vi "powerSource (1).vi"() -> ()   [LabVIEW 2013]
panel:
  out "Current, A":string
  in  "VISA Address":refnum<visa-resource-name>
  out "Voltage, V":string
  in  "Set Current":bool
  in  "Current":dbl
  in  "Set Voltage":bool
  in  "Voltage":dbl
  in  "Display Mode":enum32{"Normal", "Waveform", "Dial"}(radio)
  in  "Channel 2":bool
  out "Return":string
  in  "SCPI Command":string
  in  "Exit":bool
  in  "Read":bool
  in  "Write":bool
  in  "Connect":bool
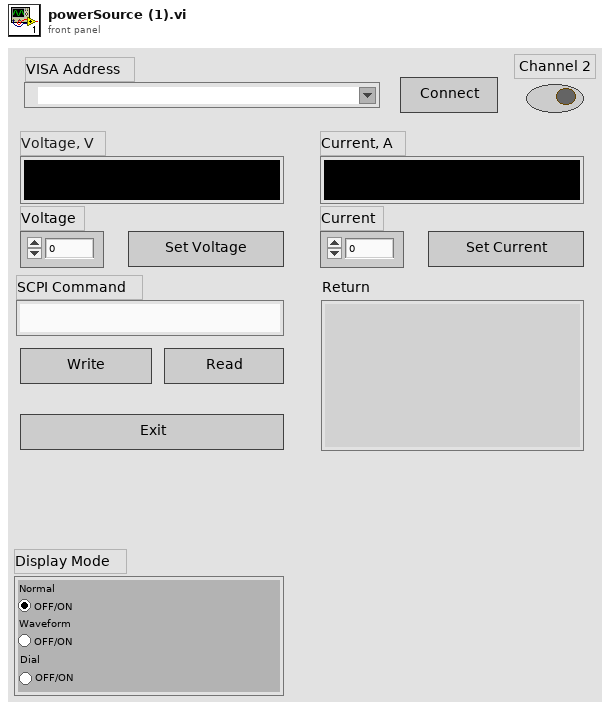
[diagram p1: front panel]
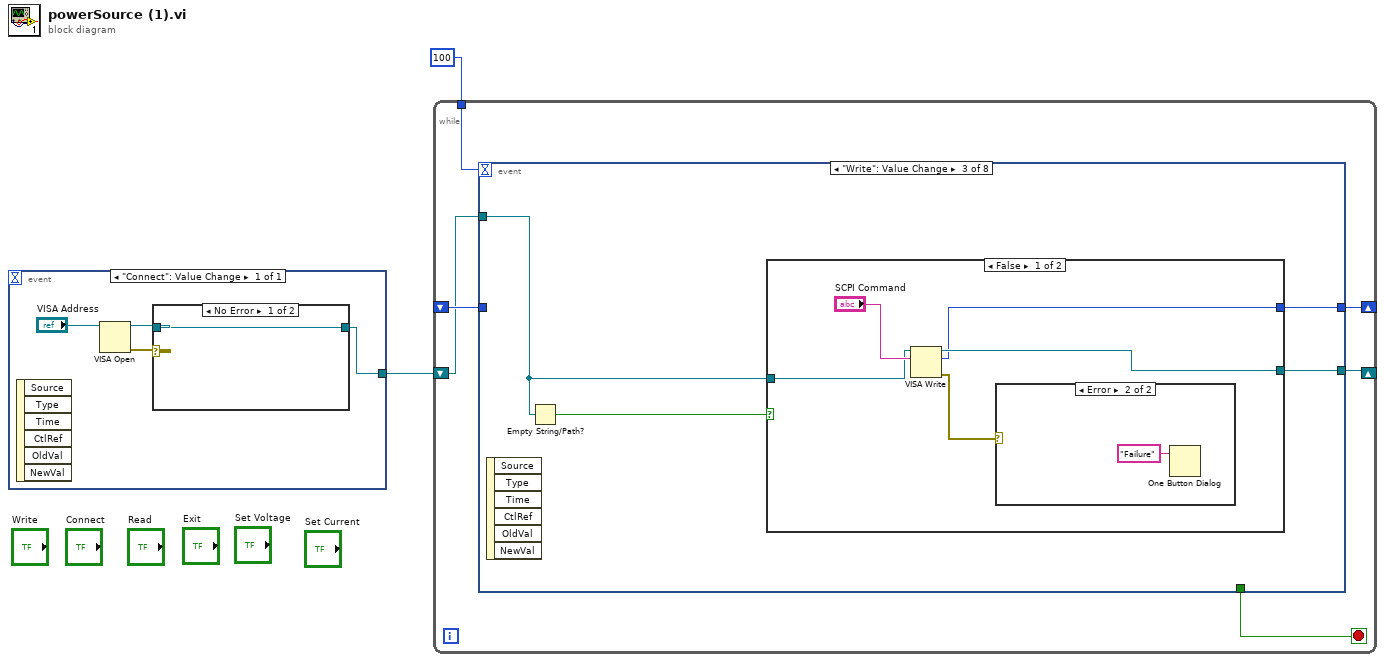
[diagram p0: block diagram]
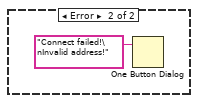
[diagram p2: hidden frame]
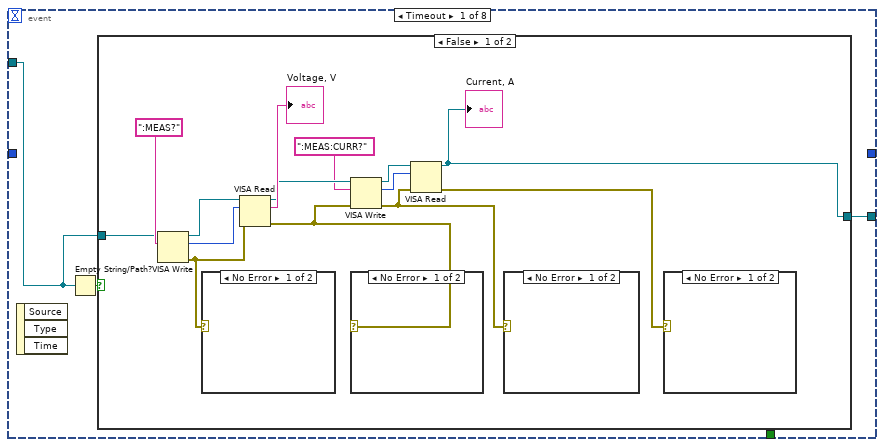
[diagram p3: hidden frame]
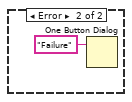
[diagram p4: hidden frame]
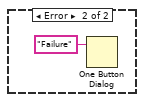
[diagram p5: hidden frame]
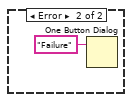
[diagram p6: hidden frame]
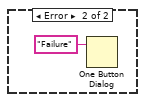
[diagram p7: hidden frame]
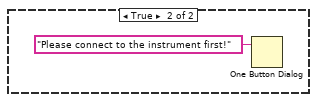
[diagram p8: hidden frame]
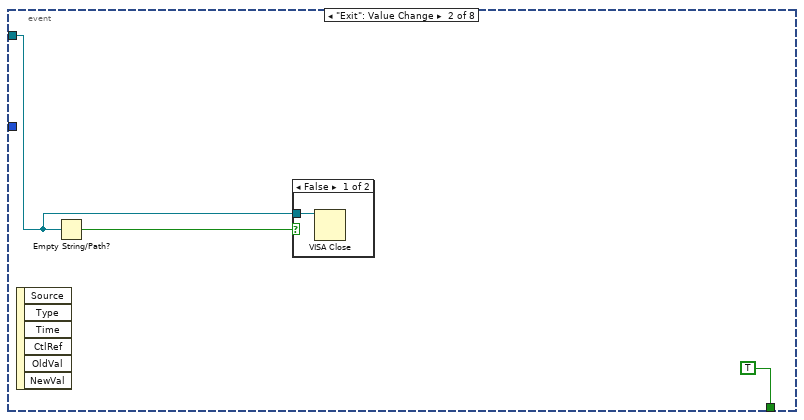
[diagram p9: hidden frame]
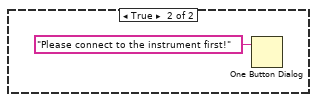
[diagram p12: hidden frame]
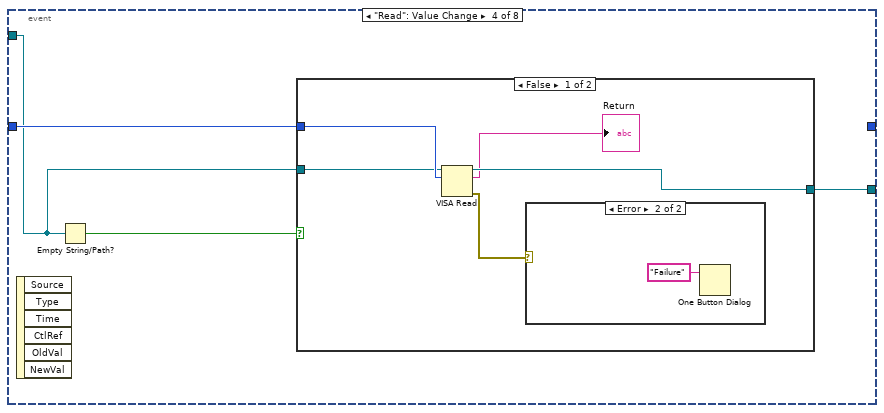
[diagram p13: hidden frame]
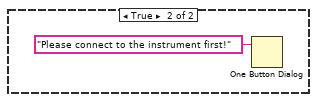
[diagram p15: hidden frame]
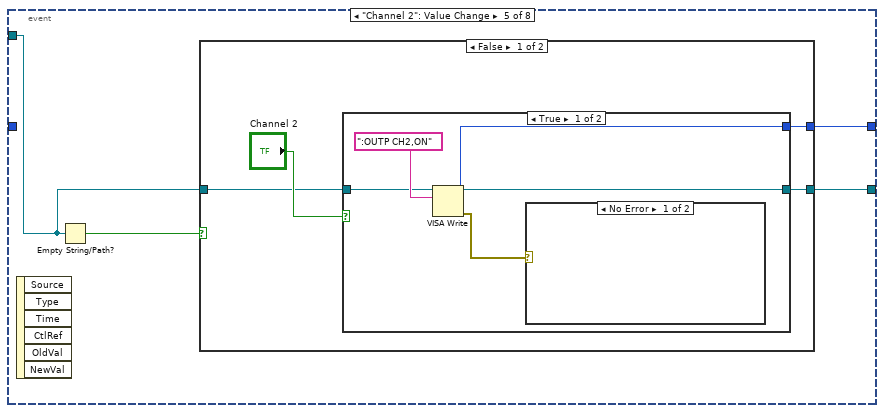
[diagram p16: hidden frame]
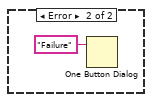
[diagram p17: hidden frame]
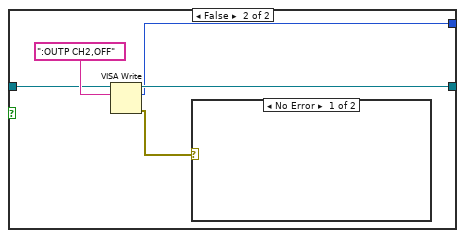
[diagram p18: hidden frame]
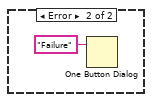
[diagram p19: hidden frame]
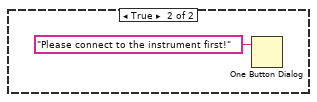
[diagram p20: hidden frame]
diagram:
  n1 = event shown="[0] \"Connect\": Value Change" {
    selector: _ -> [_]
    dyn-events: _ -> [_]
    timeout: _ -> [_]
    tunnel: [w3] -> w1
    event "Connect": Value Change {
      n2 = event-data() -> ()  [unwired: 1 in, 6 out]
      n3 = VISA Open(VISA resource name="VISA Address") -> (VISA resource name=w4:refnum<visa-resource-name>, error out=w5:errorcluster)  [unwired: 4 in]
      n4 = case shown="No Error" w5 {
        tunnel: w4 -> [w7 _]
        tunnel: [w7 _] -> w3
        frame No Error {
        }
        frame Error {
          n5 = One Button Dialog(message="Connect failed!\nInvalid address!") -> ()  [unwired: 1 in, 1 out]
        }
      }
    }
  }
  n6 = while {
    shift-right: [w14] -> _
    shift-left: w1 -> [w9]
    shift-right: [w12] -> _
    shift-left: _ -> [w11]
    tunnel: 100 -> [w10]
    stop <- w13 stop-if-true
    n7 = event shown="[2] \"Write\": Value Change" {
      selector: _ -> [_ _ _ _ _ _ _ _]
      dyn-events: _ -> [_ _ _ _ _ _ _ _]
      timeout: w10 -> [_ _ _ _ _ _ _ _]
      tunnel: [w16 _ w43 w54 w65 w86 w113 w127] -> w14
      tunnel: [_ TRUE _ _ _ _ _ _] -> w13
      tunnel: [_ _ w42 _ w64 w85 w112 w126] -> w12
      tunnel: w11 -> [_ _ _ w53 _ _ _ _]
      tunnel: w9 -> [w15 w37 w41 w52 w63 w84 w111 w125]
      event Timeout {
        n8 = event-data() -> ()  [unwired: 1 in, 3 out]
        n9 = Empty String/Path?(string/path=w15) -> (empty?=w17:bool)
        n10 = case shown="False" w17 {
          tunnel: [w18 _] -> w16
          tunnel: w15 -> [w27 _]
          frame False {
            n11 = VISA Write(VISA resource name=w27, write buffer=":MEAS?") -> (VISA resource name out=w26:refnum<visa-resource-name>, return count=w30:u32, error out=w29:errorcluster)  [unwired: 1 in]
            n12 = case shown="No Error" w29 {
              frame No Error {
              }
              frame Error {
                n13 = One Button Dialog(message="Failure") -> ()  [unwired: 1 in, 1 out]
              }
            }
            n14 = VISA Read(VISA resource name=w26, byte count=w30, error in (no error)=w29) -> (VISA resource name out=w25:refnum<visa-resource-name>, read buffer=→"Voltage, V":string, error out=w24:errorcluster)  [unwired: 1 out]
            n15 = VISA Write(VISA resource name=w25, write buffer=":MEAS:CURR?", error in (no error)=w24) -> (VISA resource name out=w22:refnum<visa-resource-name>, return count=w19:u32, error out=w21:errorcluster)
            n16 = case shown="No Error" w24 {
              frame No Error {
              }
              frame Error {
                n17 = One Button Dialog(message="Failure") -> ()  [unwired: 1 in, 1 out]
              }
            }
            n18 = VISA Read(VISA resource name=w22, byte count=w19, error in (no error)=w21) -> (VISA resource name out=w18:refnum<visa-resource-name>, error out=w20:errorcluster)  [unwired: 2 out]
            "Current, A" <- w18
            n19 = case shown="No Error" w21 {
              frame No Error {
              }
              frame Error {
                n20 = One Button Dialog(message="Failure") -> ()  [unwired: 1 in, 1 out]
              }
            }
            n21 = case shown="No Error" w20 {
              frame No Error {
              }
              frame Error {
                n22 = One Button Dialog(message="Failure") -> ()  [unwired: 1 in, 1 out]
              }
            }
          }
          frame True {
            n23 = One Button Dialog(message="Please connect to the instrument first!") -> ()  [unwired: 1 in, 1 out]
          }
        }
      }
      event "Exit": Value Change {
        n24 = event-data() -> ()  [unwired: 1 in, 6 out]
        n25 = Empty String/Path?(string/path=w37) -> (empty?=w39:bool)
        n26 = case shown="False" w39 {
          tunnel: w37 -> [w40 _]
          frame False {
            n27 = VISA Close(VISA resource name=w40) -> ()  [unwired: 1 in, 1 out]
          }
          frame True {
          }
        }
      }
      event "Write": Value Change {
        n28 = event-data() -> ()  [unwired: 1 in, 6 out]
        n29 = Empty String/Path?(string/path=w41) -> (empty?=w44:bool)
        n30 = case shown="False" w44 {
          tunnel: [w47 _] -> w43
          tunnel: [w46 _] -> w42
          tunnel: w41 -> [w45 _]
          frame False {
            n31 = VISA Write(VISA resource name=w45, write buffer="SCPI Command") -> (VISA resource name out=w47:refnum<visa-resource-name>, return count=w46:u32, error out=w48:errorcluster)  [unwired: 1 in]
            n32 = case shown="Error" w48 {
              frame No Error {
              }
              frame Error {
                n33 = One Button Dialog(message="Failure") -> ()  [unwired: 1 in, 1 out]
              }
            }
          }
          frame True {
            n34 = One Button Dialog(message="Please connect to the instrument first!") -> ()  [unwired: 1 in, 1 out]
          }
        }
      }
      event "Read": Value Change {
        n35 = event-data() -> ()  [unwired: 1 in, 6 out]
        n36 = Empty String/Path?(string/path=w52) -> (empty?=w55:bool)
        n37 = case shown="False" w55 {
          tunnel: [w60 _] -> w54
          tunnel: w53 -> [w57 _]
          tunnel: w52 -> [w56 _]
          frame False {
            n38 = VISA Read(VISA resource name=w56, byte count=w57) -> (VISA resource name out=w60:refnum<visa-resource-name>, read buffer=→"Return":string, error out=w59:errorcluster)  [unwired: 1 in, 1 out]
            n39 = case shown="Error" w59 {
              frame No Error {
              }
              frame Error {
                n40 = One Button Dialog(message="Failure") -> ()  [unwired: 1 in, 1 out]
              }
            }
          }
          frame True {
            n41 = One Button Dialog(message="Please connect to the instrument first!") -> ()  [unwired: 1 in, 1 out]
          }
        }
      }
      event "Channel 2": Value Change {
        n42 = event-data() -> ()  [unwired: 1 in, 6 out]
        n43 = Empty String/Path?(string/path=w63) -> (empty?=w66:bool)
        n44 = case shown="False" w66 {
          tunnel: [w70 _] -> w65
          tunnel: [w69 _] -> w64
          tunnel: w63 -> [w67 _]
          frame False {
            n45 = case shown="True" "Channel 2" {
              tunnel: [w73 w79] -> w70
              tunnel: [w72 w78] -> w69
              tunnel: w67 -> [w71 w77]
              frame True {
                n46 = VISA Write(VISA resource name=w71, write buffer=":OUTP CH2,ON" ("Command 2")) -> (VISA resource name out=w73:refnum<visa-resource-name>, return count=w72:u32, error out=w74:errorcluster)  [unwired: 1 in]
                n47 = case shown="No Error" w74 {
                  frame No Error {
                  }
                  frame Error {
                    n48 = One Button Dialog(message="Failure") -> ()  [unwired: 1 in, 1 out]
                  }
                }
              }
              frame False {
                n49 = VISA Write(VISA resource name=w77, write buffer=":OUTP CH2,OFF" ("Command 2")) -> (VISA resource name out=w79:refnum<visa-resource-name>, return count=w78:u32, error out=w80:errorcluster)  [unwired: 1 in]
                n50 = case shown="No Error" w80 {
                  frame No Error {
                  }
                  frame Error {
                    n51 = One Button Dialog(message="Failure") -> ()  [unwired: 1 in, 1 out]
                  }
                }
              }
            }
          }
          frame True {
            n52 = One Button Dialog(message="Please connect to the instrument first!") -> ()  [unwired: 1 in, 1 out]
          }
        }
      }
      event "Display Mode": Value Change {
        n53 = event-data() -> ()  [unwired: 1 in, 6 out]
        n54 = Empty String/Path?(string/path=w84) -> (empty?=w87:bool)
        n55 = case shown="False" w87 {
          tunnel: [w91 _] -> w86
          tunnel: [w90 _] -> w85
          tunnel: w84 -> [w88 _]
          frame False {
            n56 = case shown="\"Normal\", Default" "Display Mode" {
              tunnel: [w94 w100 w106] -> w91
              tunnel: [w93 w99 w105] -> w90
              tunnel: w88 -> [w92 w98 w104]
              frame "Normal", Default {
                n57 = VISA Write(VISA resource name=w92, write buffer=":DISP:MODE NORM" ("Command 2")) -> (VISA resource name out=w94:refnum<visa-resource-name>, return count=w93:u32, error out=w95:errorcluster)  [unwired: 1 in]
                n58 = case shown="No Error" w95 {
                  frame No Error {
                  }
                  frame Error {
                    n59 = One Button Dialog(message="Failure") -> ()  [unwired: 1 in, 1 out]
                  }
                }
              }
              frame "Waveform" {
                n60 = VISA Write(VISA resource name=w98, write buffer=":DISP:MODE WAVE" ("Command 2")) -> (VISA resource name out=w100:refnum<visa-resource-name>, return count=w99:u32, error out=w101:errorcluster)  [unwired: 1 in]
                n61 = case shown="No Error" w101 {
                  frame No Error {
                  }
                  frame Error {
                    n62 = One Button Dialog(message="Failure") -> ()  [unwired: 1 in, 1 out]
                  }
                }
              }
              frame "Dial" {
                n63 = VISA Write(VISA resource name=w104, write buffer=":DISP:MODE DIAL" ("Command 2")) -> (VISA resource name out=w106:refnum<visa-resource-name>, return count=w105:u32, error out=w107:errorcluster)  [unwired: 1 in]
                n64 = case shown="No Error" w107 {
                  frame No Error {
                  }
                  frame Error {
                    n65 = One Button Dialog(message="Failure") -> ()  [unwired: 1 in, 1 out]
                  }
                }
              }
            }
          }
          frame True {
            n66 = One Button Dialog(message="Please connect to the instrument first!") -> ()  [unwired: 1 in, 1 out]
          }
        }
      }
      event "Set Voltage": Value Change {
        n67 = event-data() -> ()  [unwired: 1 in, 6 out]
        n68 = Empty String/Path?(string/path=w111) -> (empty?=w114:bool)
        n69 = case shown="False" w114 {
          tunnel: [w121 _] -> w113
          tunnel: [w120 _] -> w112
          tunnel: w111 -> [w115 _]
          frame False {
            n70 = Number To Decimal String(number="Voltage") -> (decimal integer string=w117:string)  [unwired: 1 in]
            n71 = Concatenate Strings(":VOLT " ("Command 2"), w117) -> (w116:string)
            n72 = VISA Write(VISA resource name=w115, write buffer=w116) -> (VISA resource name out=w121:refnum<visa-resource-name>, return count=w120:u32, error out=w122:errorcluster)  [unwired: 1 in]
            n73 = case shown="No Error" w122 {
              frame No Error {
              }
              frame Error {
                n74 = One Button Dialog(message="Failure") -> ()  [unwired: 1 in, 1 out]
              }
            }
          }
          frame True {
            n75 = One Button Dialog(message="Please connect to the instrument first!") -> ()  [unwired: 1 in, 1 out]
          }
        }
      }
      event "Set Current": Value Change {
        n76 = event-data() -> ()  [unwired: 1 in, 6 out]
        n77 = Empty String/Path?(string/path=w125) -> (empty?=w128:bool)
        n78 = case shown="False" w128 {
          tunnel: [w135 _] -> w127
          tunnel: [w134 _] -> w126
          tunnel: w125 -> [w129 _]
          frame False {
            n79 = Number To Decimal String(number="Current") -> (decimal integer string=w132:string)  [unwired: 1 in]
            n80 = Concatenate Strings(":CURR " ("Command 2"), w132) -> (w131:string)
            n81 = VISA Write(VISA resource name=w129, write buffer=w131) -> (VISA resource name out=w135:refnum<visa-resource-name>, return count=w134:u32, error out=w136:errorcluster)  [unwired: 1 in]
            n82 = case shown="No Error" w136 {
              frame No Error {
              }
              frame Error {
                n83 = One Button Dialog(message="Failure") -> ()  [unwired: 1 in, 1 out]
              }
            }
          }
          frame True {
            n84 = One Button Dialog(message="Please connect to the instrument first!") -> ()  [unwired: 1 in, 1 out]
          }
        }
      }
    }
  }
